vi "CANjoiner.vi"() -> ()   [LabVIEW 2015]
panel:
  out "txtTitle":string
  in  "Language":u32
  out "待合并数组":string[][](array[string])
  out "基路径字符串":string
  out "当前格式类型":string
  out "已选格式类型":string
  in  "btnClear":bool
  in  "删除":bool
  in  "添加":bool
  in  "btnMerge":bool
  in  "ListFiles2Merge":i32[](listbox)
  out "输出结果":string
  out "txtFileInfo":string caption="File Information"
  in  "ListFolderList":i32[](listbox)
  out "基文件夹":path
  in  "btnExit":bool
  in  "btnSelectFolder":bool
  in  "FileClass":string(combo)="can" caption="文件类型："
  # "CAN离线数据合并工具"
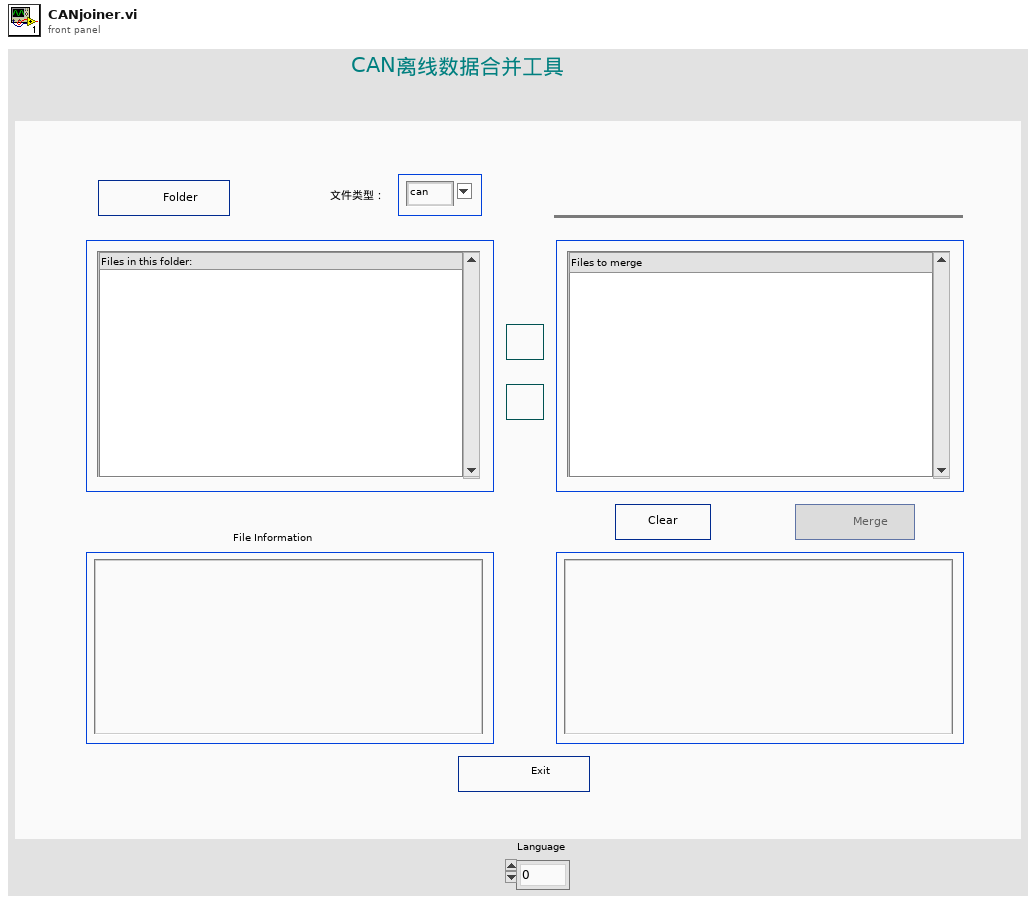
[diagram p1: front panel]
types:
  T1 = enum8{"Enabled", "Disabled", "Disabled and Grayed Out"}
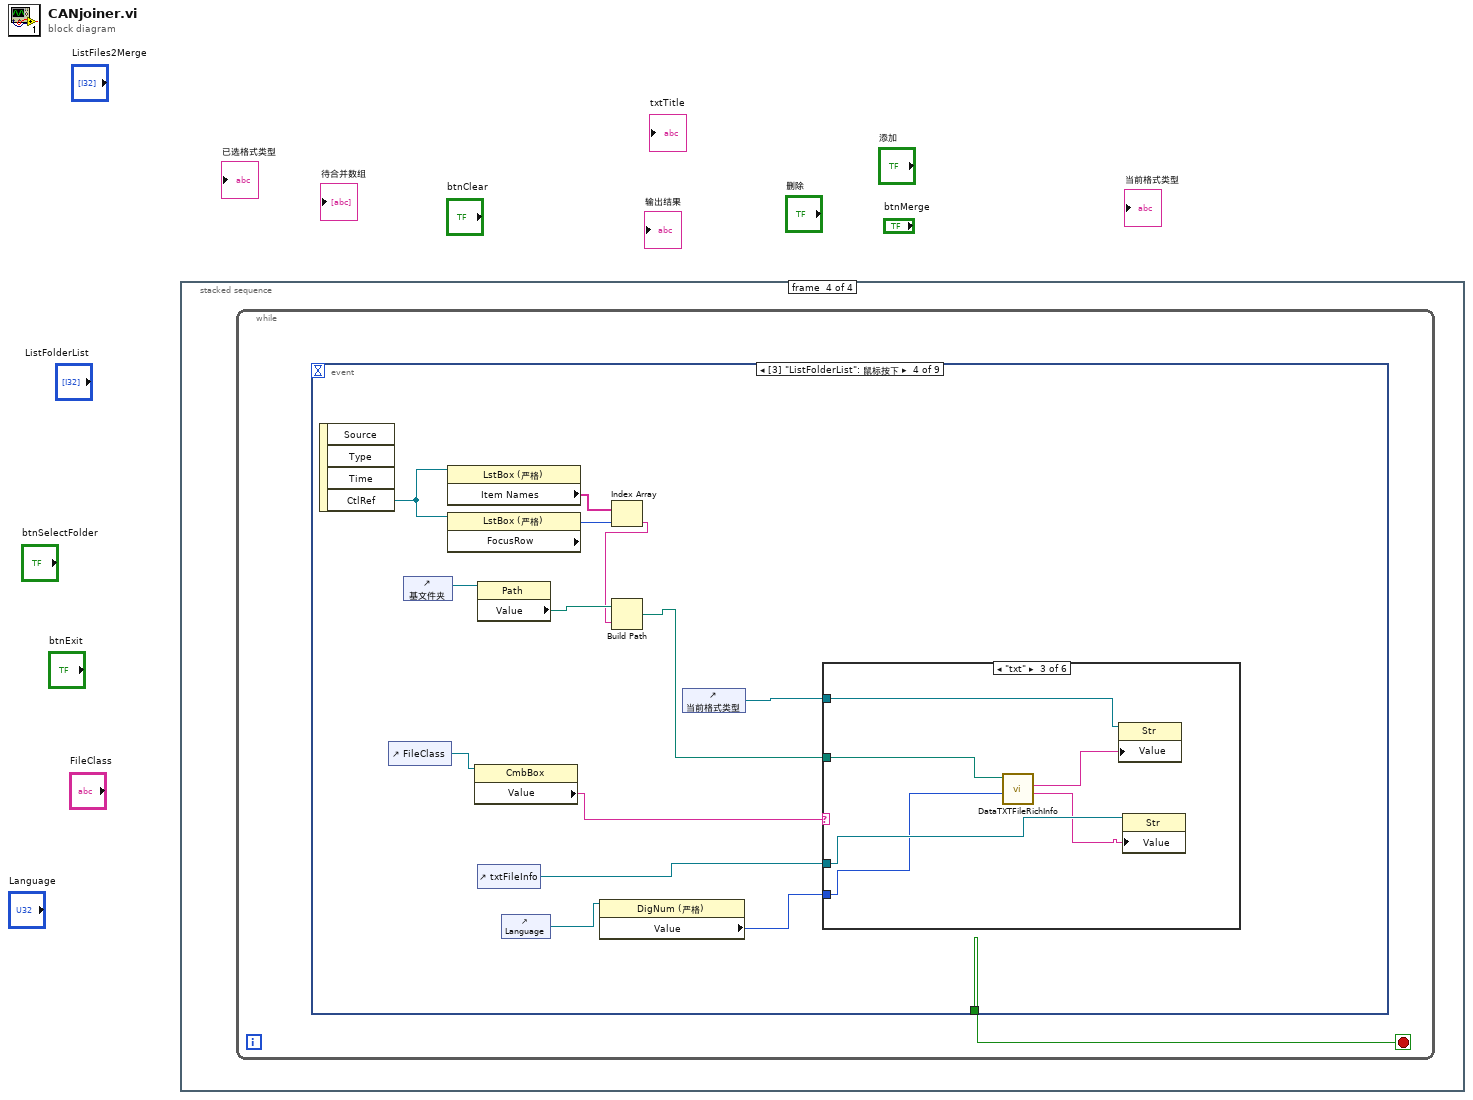
[diagram p0: block diagram]
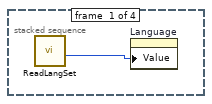
[diagram p2: hidden frame]
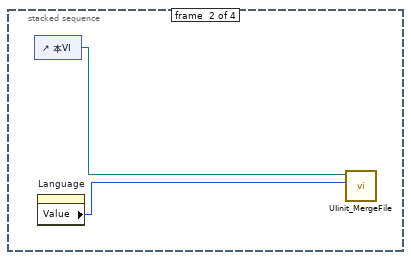
[diagram p3: hidden frame]
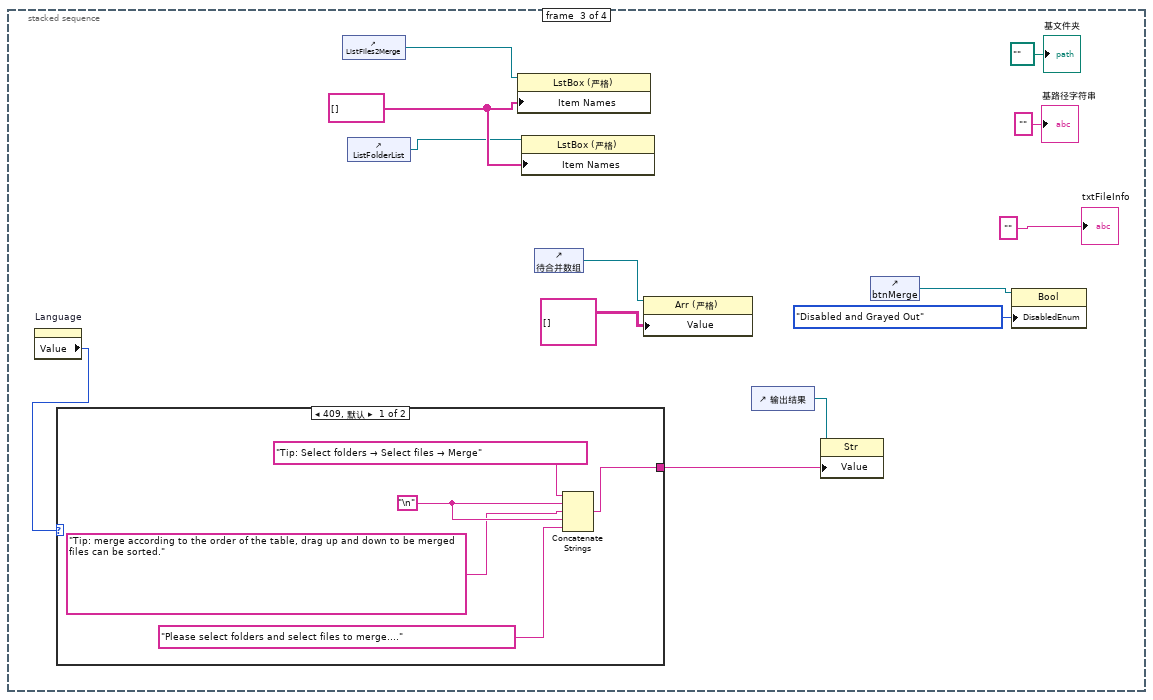
[diagram p4: hidden frame]
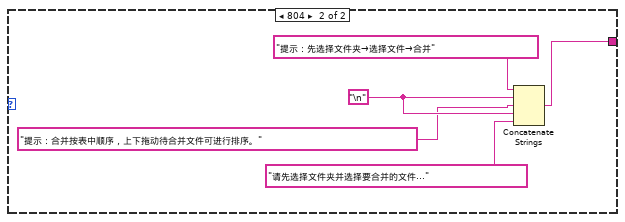
[diagram p5: hidden frame]
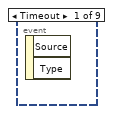
[diagram p6: hidden frame]
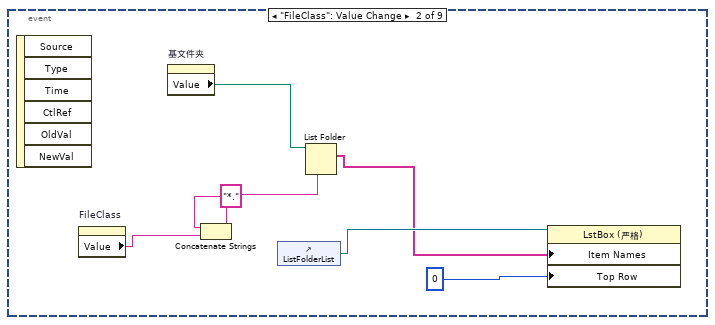
[diagram p7: hidden frame]
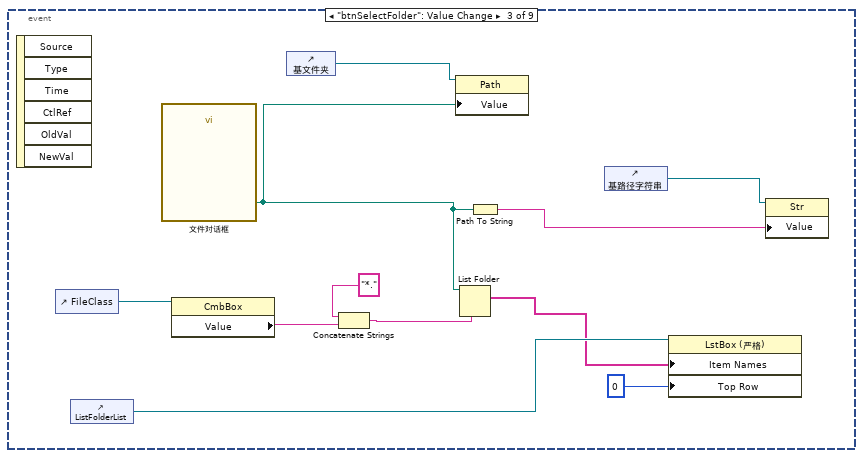
[diagram p8: hidden frame]
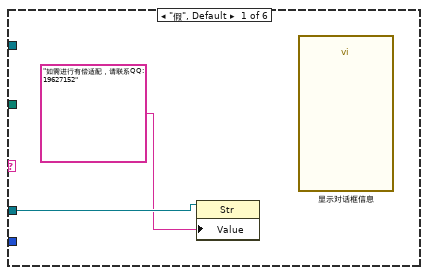
[diagram p9: hidden frame]
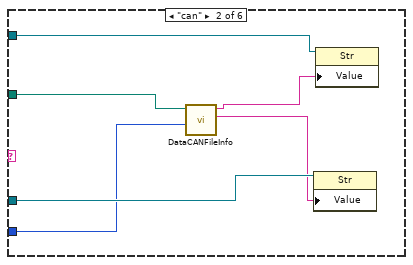
[diagram p10: hidden frame]
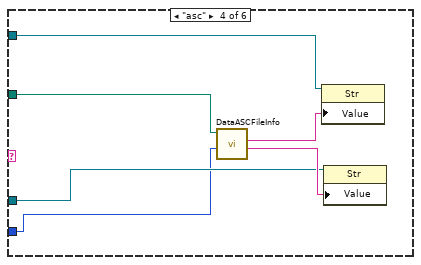
[diagram p11: hidden frame]
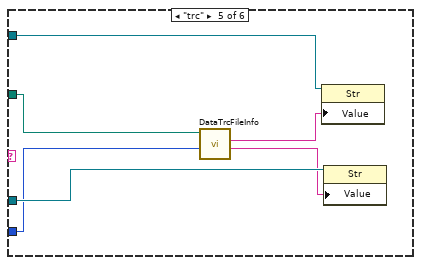
[diagram p12: hidden frame]
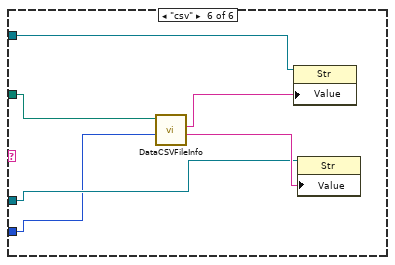
[diagram p13: hidden frame]
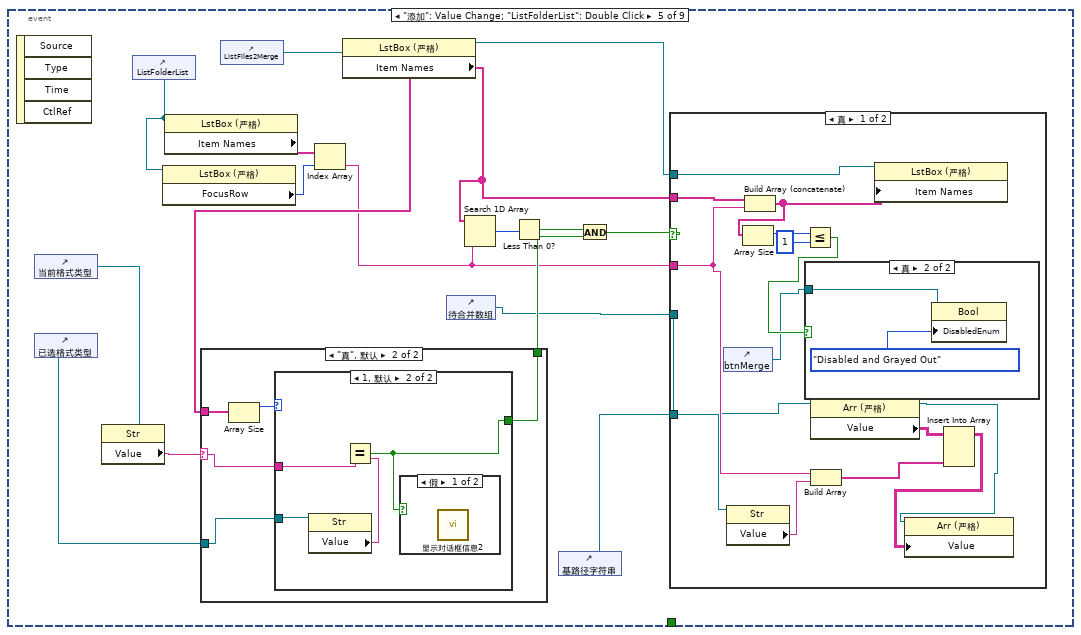
[diagram p14: hidden frame]
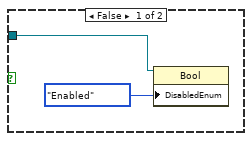
[diagram p15: hidden frame]
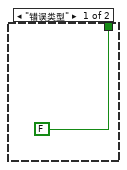
[diagram p17: hidden frame]
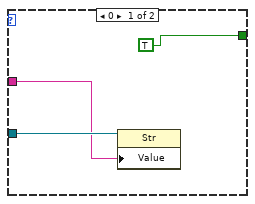
[diagram p18: hidden frame]
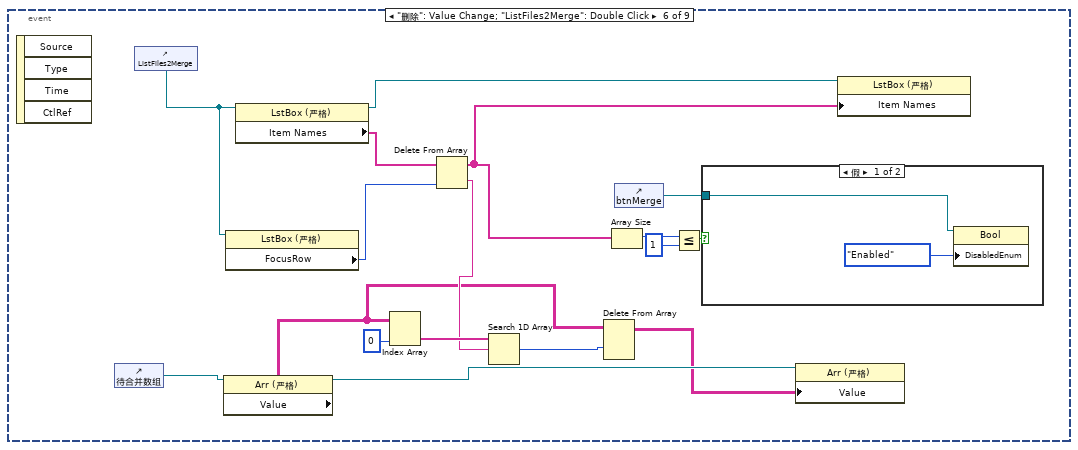
[diagram p20: hidden frame]
diagram:
  n1 = stacked-sequence {
    frame #0 {
      n2 = call "ReadLangSet.vi"() -> ("Language"=w1:u32)  [unwired: 11 in]
      n3 = property on="Language" class="DigNum (严格)"("Value"=w1) -> ()  [unwired: 2 in, 2 out]
    }
    frame #1 {
      n4 = control-ref of="本VI"() -> (w3:refnum<vi>)
      n5 = property on="Language" class="DigNum (严格)"() -> ("Value"=w2:u32)  [unwired: 2 in, 2 out]
      n6 = call "UIinit_MergeFile.vi"("Language"=w2, "VI输入"=w3) -> ()  [unwired: 10 in]
    }
    frame #2 {
      w9 = string[] []
      n7 = property on="Language" class="DigNum (严格)"() -> ("Value"=w4:u32)  [unwired: 2 in, 2 out]
      n8 = case shown="409, 默认" w4 {
        tunnel: [w17 w25] -> w14
        frame 409, Default {
          w19 = "\n"
          n9 = Concatenate Strings("Tip: Select folders → Select files → Merge" ("值"), w19, "Tip: merge according to the order of the table, drag up and down to be merged files can be sorted." ("值"), w19, "Please select folders and select files to merge...." ("值")) -> (w17:string)
        }
        frame 804 {
          w23 = "\n"
          n10 = Concatenate Strings("提示：先选择文件夹→选择文件→合并" ("值"), w23, "提示：合并按表中顺序，上下拖动待合并文件可进行排序。" ("值"), w23, "请先选择文件夹并选择要合并的文件..." ("值")) -> (w25:string)
        }
      }
      n11 = control-ref of="ListFiles2Merge"() -> (w16:refnum<vi>)
      n12 = control-ref of="ListFolderList"() -> (w8:refnum<vi>)
      n13 = property class="LstBox (严格)"(reference=w16, "Item Names"=w9) -> ()  [unwired: 1 in, 2 out]
      n14 = property class="LstBox (严格)"(reference=w8, "Item Names"=w9) -> ()  [unwired: 1 in, 2 out]
      n15 = control-ref of="待合并数组"() -> (w13:refnum<vi>)
      n16 = property class="Arr (严格)"(reference=w13, "Value"=string[][] [] ("待合并数组")) -> ()  [unwired: 1 in, 2 out]
      n17 = control-ref of="输出结果"() -> (w15:refnum<vi>)
      n18 = property class="Str"(reference=w15, "Value"=w14) -> ()  [unwired: 1 in, 2 out]
      n19 = control-ref of="btnMerge"() -> (w6:refnum<vi>)
      n20 = property class="Bool"(reference=w6, "DisabledEnum"=T1."Disabled and Grayed Out" ("禁用")) -> ()  [unwired: 1 in, 2 out]
      "基文件夹" <- path "" ("基文件夹")
      "基路径字符串" <- "" ("基路径字符串")
      "txtFileInfo" <- "" ("文件信息")
    }
    frame #3 {
      n21 = while {
        stop <- w27 stop-if-true
        n22 = event shown="[3] \"ListFolderList\": 鼠标按下" {
          selector: _ -> [_ _ _ _ _ _ _ _ _]
          dyn-events: _ -> [_ _ _ _ _ _ _ _ _]
          timeout: _ -> [_ _ _ _ _ _ _ _ _]
          tunnel: [_ _ _ _ _ _ _ TRUE _] -> w27
          event Timeout {
            n23 = event-data() -> ()  [unwired: 1 in, 2 out]
          }
          event "FileClass": Value Change {
            n24 = event-data() -> ()  [unwired: 1 in, 6 out]
            n25 = property on="FileClass" class="CmbBox"() -> ("Value"=w31:string)  [unwired: 2 in, 2 out]
            n26 = property on="基文件夹" class="Path"() -> ("Value"=w32:path)  [unwired: 2 in, 2 out]
            n27 = Concatenate Strings("*." ("字符串"), w31) -> (w34:string)
            n28 = control-ref of="ListFolderList"() -> (w30:refnum<vi>)
            n29 = List Folder(path=w32, pattern=w34) -> (filenames=w29:string[])  [unwired: 2 in, 3 out]
            n30 = property class="LstBox (严格)"(reference=w30, "Item Names"=w29, "Top Row"=0 ("选中行")) -> ()  [unwired: 1 in, 2 out]
          }
          event "btnSelectFolder": Value Change {
            n31 = event-data() -> ()  [unwired: 1 in, 6 out]
            n32 = control-ref of="FileClass"() -> (w42:refnum<vi>)
            n33 = control-ref of="ListFolderList"() -> (w37:refnum<vi>)
            n34 = call "文件对话框"() -> ("selected path"=w40:path)  [unwired: 12 in, 3 out]
            n35 = property class="CmbBox"(reference=w42) -> ("Value"=w43:string)  [unwired: 1 in, 2 out]
            n36 = control-ref of="基文件夹"() -> (w41:refnum<vi>)
            n37 = Concatenate Strings("*." ("字符串"), w43) -> (w45:string)
            n38 = property class="Path"(reference=w41, "Value"=w40) -> ()  [unwired: 1 in, 2 out]
            n39 = List Folder(path=w40, pattern=w45) -> (filenames=w36:string[])  [unwired: 2 in, 3 out]
            n40 = Path To String(path=w40) -> (string=w38:string)
            n41 = control-ref of="基路径字符串"() -> (w39:refnum<vi>)
            n42 = property class="LstBox (严格)"(reference=w37, "Item Names"=w36, "Top Row"=0 ("选中行")) -> ()  [unwired: 1 in, 2 out]
            n43 = property class="Str"(reference=w39, "Value"=w38) -> ()  [unwired: 1 in, 2 out]
          }
          event "ListFolderList": Mouse Down {
            n44 = event-data() -> ("CtlRef"=w56:refnum<vi>)  [unwired: 1 in, 3 out]
            n45 = control-ref of="FileClass"() -> (w49:refnum<vi>)
            n46 = control-ref of="基文件夹"() -> (w55:refnum<vi>)
            n47 = property class="LstBox (严格)"(reference=w56) -> ("Item Names"=w58:string[])  [unwired: 1 in, 2 out]
            n48 = property class="LstBox (严格)"(reference=w56) -> ("FocusRow"=w57:i32)  [unwired: 1 in, 2 out]
            n49 = property class="CmbBox"(reference=w49) -> ("Value"=w48:string)  [unwired: 1 in, 2 out]
            n50 = property class="Path"(reference=w55) -> ("Value"=w54:path)  [unwired: 1 in, 2 out]
            n51 = control-ref of="txtFileInfo"() -> (w51:refnum<vi>)
            n52 = control-ref of="Language"() -> (w47:refnum<vi>)
            n53 = property class="DigNum (严格)"(reference=w47) -> ("Value"=w46:u32)  [unwired: 1 in, 2 out]
            n54 = Index Array(array=w58, index=w57) -> (element=w53:string)
            n55 = Build Path(base path=w54, name or relative path=w53) -> (appended path=w52:path)
            n56 = control-ref of="当前格式类型"() -> (w50:refnum<vi>)
            n57 = case shown="\"txt\"" w48 {
              tunnel: w52 -> [_ w66 w67 w78 w82 w90]
              tunnel: w51 -> [w60 w65 w71 w74 w83 w87]
              tunnel: w50 -> [_ w63 w72 w77 w84 w86]
              tunnel: w46 -> [_ w61 w68 w73 w81 w85]
              frame "假", Default {
                n58 = property class="Str"(reference=w60, "Value"="如需进行有偿适配，请联系QQ:19627152") -> ()  [unwired: 1 in, 2 out]
                n59 = call "显示对话框信息"() -> ()  [unwired: 10 in, 2 out]
              }
              frame "can" {
                n60 = call "DataCANFileInfo.vi"("Language"=w61, "file path (dialog if empty)"=w66) -> ("FileInfo"=w64:string, "文件类型"=w62:string)  [unwired: 7 in, 1 out]
                n61 = property class="Str"(reference=w65, "Value"=w64) -> ()  [unwired: 1 in, 2 out]
                n62 = property class="Str"(reference=w63, "Value"=w62) -> ()  [unwired: 1 in, 2 out]
              }
              frame "txt" {
                n63 = call "DataTXTFileRichInfo.vi"("Language"=w68, "file path (dialog if empty)"=w67) -> ("FileInfo"=w70:string, "文件类型"=w69:string)  [unwired: 7 in, 1 out]
                n64 = property class="Str"(reference=w72, "Value"=w69) -> ()  [unwired: 1 in, 2 out]
                n65 = property class="Str"(reference=w71, "Value"=w70) -> ()  [unwired: 1 in, 2 out]
              }
              frame "asc" {
                n66 = call "DataASCFileInfo.vi"("Language"=w73, "file path (dialog if empty)"=w78) -> ("FileInfo"=w75:string, "文件类型"=w76:string)  [unwired: 7 in, 1 out]
                n67 = property class="Str"(reference=w77, "Value"=w76) -> ()  [unwired: 1 in, 2 out]
                n68 = property class="Str"(reference=w74, "Value"=w75) -> ()  [unwired: 1 in, 2 out]
              }
              frame "trc" {
                n69 = call "DataTrcFileInfo.vi"("Language"=w81, "file path (dialog if empty)"=w82) -> ("FileInfo"=w79:string, "文件类型"=w80:string)  [unwired: 7 in, 1 out]
                n70 = property class="Str"(reference=w84, "Value"=w80) -> ()  [unwired: 1 in, 2 out]
                n71 = property class="Str"(reference=w83, "Value"=w79) -> ()  [unwired: 1 in, 2 out]
              }
              frame "csv" {
                n72 = call "DataCSVFileInfo.vi"("Language"=w85, "file path (dialog if empty)"=w90) -> ("FileInfo"=w88:string, "文件类型"=w89:string)  [unwired: 7 in, 1 out]
                n73 = property class="Str"(reference=w86, "Value"=w89) -> ()  [unwired: 1 in, 2 out]
                n74 = property class="Str"(reference=w87, "Value"=w88) -> ()  [unwired: 1 in, 2 out]
              }
            }
          }
          event "添加": Value Change; "ListFolderList": Double Click {
            n75 = event-data() -> ()  [unwired: 1 in, 4 out]
            n76 = control-ref of="当前格式类型"() -> (w98:refnum<vi>)
            n77 = control-ref of="已选格式类型"() -> (w99:refnum<vi>)
            n78 = property class="Str"(reference=w98) -> ("Value"=w97:string)  [unwired: 1 in, 2 out]
            n79 = control-ref of="ListFolderList"() -> (w104:refnum<vi>)
            n80 = property class="LstBox (严格)"(reference=w104) -> ("FocusRow"=w105:i32)  [unwired: 1 in, 2 out]
            n81 = property class="LstBox (严格)"(reference=w104) -> ("Item Names"=w106:string[])  [unwired: 1 in, 2 out]
            n82 = control-ref of="ListFiles2Merge"() -> (w100:refnum<vi>)
            n83 = Index Array(array=w106, index=w105) -> (element=w94:string)
            n84 = property class="LstBox (严格)"(reference=w100) -> (reference out=w96:refnum<vi>, "Item Names"=w95:string[])  [unwired: 1 in, 1 out]
            n85 = case shown="\"真\", 默认" w97 {
              selector: w97 -> [_ w127]
              tunnel: w95 -> [_ w131]
              tunnel: [FALSE w129] -> w101
              tunnel: w99 -> [_ w128]
              frame "错误类型" {
              }
              frame "真", Default {
                n86 = Array Size(array=w131) -> (size(s)=w130:i32)
                n87 = case shown="1, 默认" w130 {
                  tunnel: [TRUE w137] -> w129
                  tunnel: w128 -> [w133 w136]
                  tunnel: w127 -> [w132 w135]
                  frame 0 {
                    n88 = property on="属性节点" class="Str"(reference=w133, "Value"=w132) -> ()  [unwired: 1 in, 2 out]
                  }
                  frame 1, Default {
                    n89 = property on="属性节点" class="Str"(reference=w136) -> ("Value"=w138:string)  [unwired: 1 in, 2 out]
                    n90 = Equal?(x=w135, y=w138) -> (x = y?=w137:bool)
                    n91 = case shown="假" w137 {
                      frame False {
                        n92 = call "显示对话框信息2"() -> ()  [unwired: 10 in, 2 out]
                      }
                      frame True {
                      }
                    }
                  }
                }
              }
            }
            n93 = control-ref of="待合并数组"() -> (w91:refnum<vi>)
            n94 = Search 1D Array(1D array=w95, element=w94) -> (index of element=w103:i32)  [unwired: 1 in]
            n95 = Less Than 0?(x=w103) -> (x < 0?=w102:bool)
            n96 = control-ref of="基路径字符串"() -> (w92:refnum<vi>)
            n97 = And(x=w102, y=w101) -> (x .and. y?=w93:bool)
            n98 = case shown="真" w93 {
              tunnel: w94 -> [w119 _]
              tunnel: w95 -> [w121 _]
              tunnel: w96 -> [w120 _]
              tunnel: w92 -> [w118 _]
              tunnel: w91 -> [w115 _]
              frame True {
                n99 = control-ref of="btnMerge"() -> (w107:refnum<vi>)
                n100 = property class="Str"(reference=w118) -> ("Value"=w117:string)  [unwired: 1 in, 2 out]
                n101 = Build Array (concatenate)(w121, w119) -> (w109:string[])
                n102 = Array Size(array=w109) -> (size(s)=w111:i32)
                n103 = Less Or Equal?(x=w111, y=1) -> (x <= y?=w108:bool)
                n104 = case shown="真" w108 {
                  tunnel: w107 -> [w122 w124]
                  frame False {
                    n105 = property class="Bool"(reference=w122, "DisabledEnum"=T1."Enabled" ("禁用")) -> ()  [unwired: 1 in, 2 out]
                  }
                  frame True {
                    n106 = property class="Bool"(reference=w124, "DisabledEnum"=T1."Disabled and Grayed Out" ("禁用")) -> ()  [unwired: 1 in, 2 out]
                  }
                }
                n107 = property class="Arr (严格)"(reference=w115) -> (reference out=w113:refnum<vi>, "Value"=w114:string[][])  [unwired: 1 in, 1 out]
                n108 = Build Array(w119, w117) -> (w116:string[])
                n109 = property class="LstBox (严格)"(reference=w120, "Item Names"=w109) -> ()  [unwired: 1 in, 2 out]
                n110 = Insert Into Array(array=w114, new element=w116) -> (w112:string[][])  [unwired: 2 in]
                n111 = property class="Arr (严格)"(reference=w113, "Value"=w112) -> ()  [unwired: 1 in, 2 out]
              }
              frame False {
              }
            }
          }
          event "删除": Value Change; "ListFiles2Merge": Double Click {
            n112 = event-data() -> ()  [unwired: 1 in, 4 out]
            n113 = control-ref of="待合并数组"() -> (w151:refnum<vi>)
            n114 = control-ref of="ListFiles2Merge"() -> (w152:refnum<vi>)
            n115 = property class="Arr (严格)"(reference=w151) -> (reference out=w145:refnum<vi>, "Value"=w147:string[][])  [unwired: 1 in, 1 out]
            n116 = property class="LstBox (严格)"(reference=w152) -> ("FocusRow"=w153:i32)  [unwired: 1 in, 2 out]
            n117 = property class="LstBox (严格)"(reference=w152) -> (reference out=w154:refnum<vi>, "Item Names"=w155:string[])  [unwired: 1 in, 1 out]
            n118 = Index Array(array=w147, index (col)=0 ("禁用的索引 (列)")) -> (element=w149:string[])  [unwired: 1 in]
            n119 = Delete From Array(array=w155, index=w153) -> (deleted portion=w148:string, array with subset deleted=w143:string[])  [unwired: 1 in]
            n120 = Search 1D Array(1D array=w149, element=w148) -> (index of element=w146:i32)  [unwired: 1 in]
            n121 = Delete From Array(array=w147, index (row)=w146) -> (array with subset deleted=w144:string[][])  [unwired: 2 in, 1 out]
            n122 = Array Size(array=w143) -> (size(s)=w142:i32)
            n123 = control-ref of="btnMerge"() -> (w139:refnum<vi>)
            n124 = Less Or Equal?(x=w142, y=1) -> (x <= y?=w140:bool)
            n125 = case shown="假" w140 {
              tunnel: w139 -> [w156 w158]
              frame False {
                n126 = property class="Bool"(reference=w156, "DisabledEnum"=T1."Enabled" ("禁用")) -> ()  [unwired: 1 in, 2 out]
              }
              frame True {
                n127 = property class="Bool"(reference=w158, "DisabledEnum"=T1."Disabled and Grayed Out" ("禁用")) -> ()  [unwired: 1 in, 2 out]
              }
            }
            n128 = property class="Arr (严格)"(reference=w145, "Value"=w144) -> ()  [unwired: 1 in, 2 out]
            n129 = property class="LstBox (严格)"(reference=w154, "Item Names"=w143) -> ()  [unwired: 1 in, 2 out]
          }
          event "btnClear": Value Change {
            n130 = event-data() -> ()  [unwired: 1 in, 6 out]
            n131 = control-ref of="待合并数组"() -> (w163:refnum<vi>)
            n132 = control-ref of="ListFiles2Merge"() -> (w164:refnum<vi>)
            n133 = property class="Arr (严格)"(reference=w163, "Value"=string[][] [] ("值")) -> ()  [unwired: 1 in, 2 out]
            n134 = property class="LstBox (严格)"(reference=w164, "Item Names"=string[] []) -> ()  [unwired: 1 in, 2 out]
            n135 = control-ref of="btnMerge"() -> (w160:refnum<vi>)
            n136 = property class="Bool"(reference=w160, "DisabledEnum"=T1."Disabled and Grayed Out" ("禁用")) -> ()  [unwired: 1 in, 2 out]
          }
          event "btnExit": Value Change; Panel Close {
            n137 = event-data() -> ()  [unwired: 1 in, 3 out]
            n138 = control-ref of="本VI"() -> (w168:refnum<vi>)
            n139 = invoke class="VI" method="FP.Close"(reference=w168) -> (reference out=w167:refnum<vi>, error out=w166:errorcluster)  [unwired: 2 in, 1 out]
            n140 = Close Reference(reference=w167, error in (no error)=w166) -> ()  [unwired: 1 out]
          }
          event "btnMerge": Value Change {
            n141 = event-data() -> ()  [unwired: 1 in, 6 out]
            n142 = stacked-sequence {
              seq-local: [w171 _ _] -> [_ w176 _]
              seq-local: [w170 _ _] -> [_ w175 _]
              frame #0 {
                n143 = control-ref of="ListFiles2Merge"() -> (w174:refnum<vi>)
                n144 = control-ref of="待合并数组"() -> (w173:refnum<vi>)
                n145 = control-ref of="已选格式类型"() -> (w172:refnum<vi>)
                n146 = control-ref of="输出结果"() -> (w170:refnum<vi>)
                n147 = call "MergeFiles.vi"("输出结果"=w170, "SelectedFormat"=w172, "FileList"=w174, "FilesArry"=w173) -> ("Path"=w171:path)  [unwired: 7 in]
              }
              frame #1 {
                n148 = call <vilib>:"Is Path and Not Empty.vi"("path"=w176) -> ("Is Path and Not Empty?"=w177:bool)  [unwired: 4 in]
                n149 = case shown="真" w177 {
                  tunnel: w176 -> [_ w184]
                  tunnel: w175 -> [_ w178]
                  frame False {
                  }
                  frame True {
                    n150 = Path To String(path=w184) -> (string=w180:string)
                    n151 = Concatenate Strings("合并成功！", "\n", "文件已保存至：", w180) -> (w179:string)
                    n152 = property class="Str"(reference=w178, "Value"=w179) -> ()  [unwired: 1 in, 2 out]
                  }
                }
              }
              frame #2 {
                n153 = control-ref of="FileClass"() -> (w186:refnum<vi>)
                n154 = control-ref of="ListFolderList"() -> (w185:refnum<vi>)
                n155 = property class="CmbBox"(reference=w186) -> ("Value"=w191:string)  [unwired: 1 in, 2 out]
                n156 = control-ref of="基文件夹"() -> (w188:refnum<vi>)
                n157 = property class="Path"(reference=w188) -> ("Value"=w187:path)  [unwired: 1 in, 2 out]
                n158 = Concatenate Strings("*." ("字符串"), w191) -> (w193:string)
                n159 = List Folder(path=w187, pattern=w193) -> (filenames=w190:string[])  [unwired: 2 in, 3 out]
                n160 = property class="LstBox (严格)"(reference=w185, "Item Names"=w190, "Top Row"=0 ("选中行")) -> ()  [unwired: 1 in, 2 out]
              }
            }
          }
        }
      }
    }
  }
